vi "SendCommand.vi"(8 "error in (no error)":errorcluster, 11 "TCPComm in":refnum<class "TCPCommClass.lvclass">) -> (0 "error out":errorcluster, 3 "TCPComm out":refnum<class "TCPCommClass.lvclass">)   [LabVIEW 2020, in "TCPCommClass.lvclass"]
uses:
  TCPCommClass.lvclass
  C:/GEECS/Developers Version/source/Device Drivers/Picomotor8742/SupportLibs/ASCIICommClass/ASCIICommClass.lvclass
  TCPCommClass.lvclass/TCPCommClass.ctl
panel:
  in  "Initial byte timeout ms (1000)":i32=10
  in  "old tcp":bool
  # "This device sends nothing back after a command. so dont wait for something"
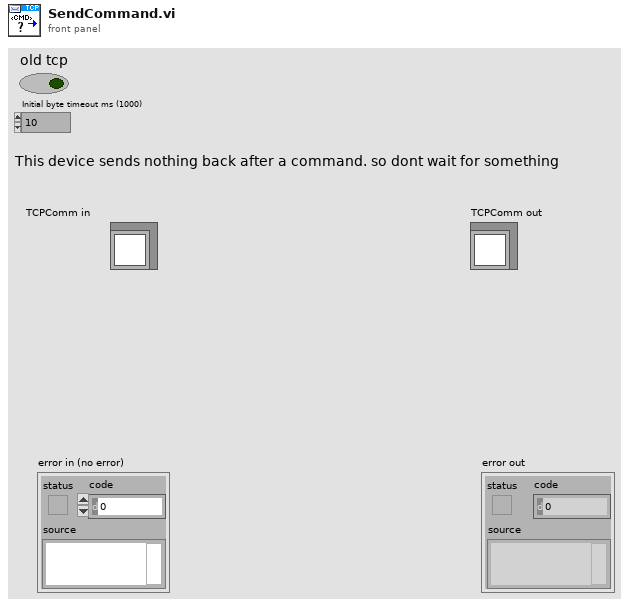
[diagram p1: front panel]
types:
  T1 = enum16{"Standard", "Buffered", "CRLF", "Immediate"}
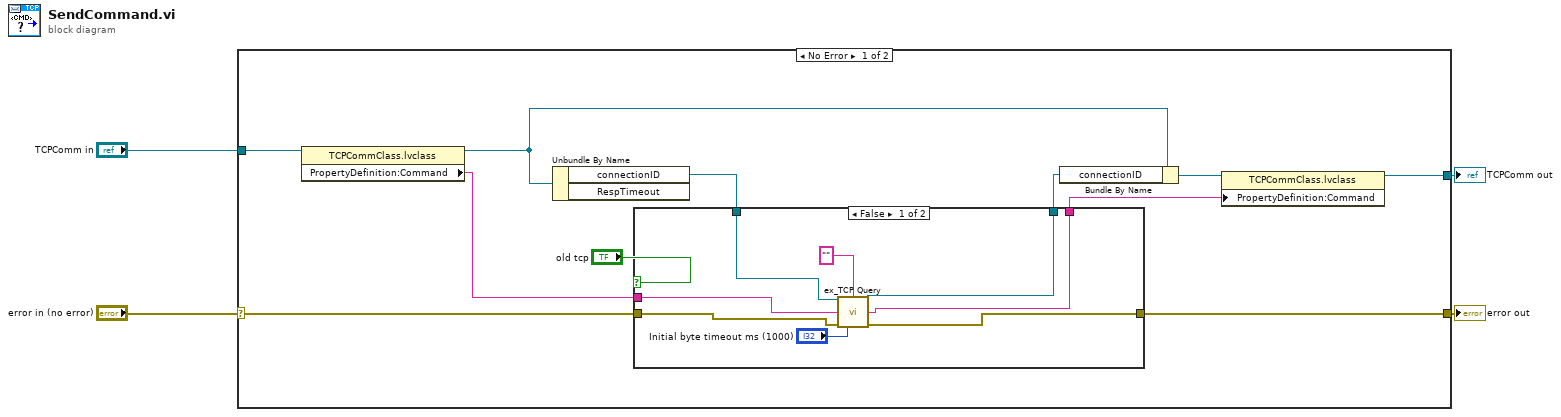
[diagram p0: block diagram]
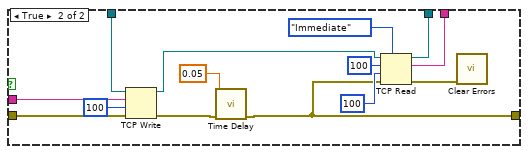
[diagram p2: hidden frame]
diagram:
  n1 = case shown="No Error" "error in (no error)" {
    selector: "error in (no error)" -> [w15 w39]
    tunnel: [w6 w39] -> w3
    tunnel: [w9 w38] -> w1
    tunnel: "TCPComm in" -> [w13 w38]
    frame No Error {
      n2 = property class="TCPCommClass.lvclass"(reference=w13) -> (reference out=w12:refnum<class "TCPCommClass.lvclass">, "PropertyDefinition:Command"=w11:string)  [unwired: 1 in, 1 out]
      n3 = Unbundle By Name(w12) -> ("connectionID"=w14:refnum<k5>)  [unwired: 1 out]
      n4 = case shown="False" "old tcp" {
        tunnel: w15 -> [w21 w37]
        tunnel: w14 -> [w23 w36]
        tunnel: w11 -> [w22 w35]
        tunnel: [w18 w32] -> w8
        tunnel: [w19 w28] -> w7
        tunnel: [w20 w24] -> w6
        frame False {
          n5 = call "ex_TCP Query.vi"("TCP Network Connection in"=w23, "Termination character"="", "Query string"=w22, "error in (no error)"=w21, "Initial byte timeout ms (1000)"="Initial byte timeout ms (1000)") -> ("TCP Network Connection out"=w18:refnum<k5>, "Message data out"=w19:string, "error out"=w20:errorcluster)  [unwired: 7 in, 1 out]
        }
        frame True {
          n6 = TCP Write(connection ID=w36, data in=w35, error in (no error)=w37, 9:100 ("bytes to read")) -> (connection ID out=w33:refnum<k5>, error out=w25:errorcluster)  [unwired: 1 out]
          n7 = call "Time Delay"("error in (no error)"=w25, "Delay Time (s)"=0.05) -> ("error out"=w24:errorcluster)  [unwired: 9 in]
          n8 = TCP Read(connection ID=w33, bytes to read=100, error in (no error)=w24, 7:T1."Immediate" ("mode (standard)"), 9:100 ("timeout ms (25000)")) -> (connection ID out=w32:refnum<k5>, data out=w28:string, error out=w29:errorcluster)
          n9 = call <vilib>:"Clear Errors.vi"("error in (no error)"=w29) -> ()  [unwired: 5 in, 2 out]
        }
      }
      n10 = Bundle By Name(cluster=w12, "connectionID"=w8) -> (w10:refnum<class "TCPCommClass.lvclass">)
      n11 = property class="TCPCommClass.lvclass"(reference=w10, "PropertyDefinition:Command"=w7) -> (reference out=w9:refnum<class "TCPCommClass.lvclass">)  [unwired: 1 in, 1 out]
    }
    frame Error {
    }
  }
  "error out" <- w3
  "TCPComm out" <- w1
